vi "Get Set Operation.vi"(7 "Type":T1, 9 "String Operation":string, 11 "Numeric Operation":string) -> (2 "Operation":string)   [LabVIEW 2016]
uses:
  <vilib>/Utility/Data Type/Type Definitions/Data Type.ctl
  <vilib>/Utility/Data Type/NI_Data Type.lvlib
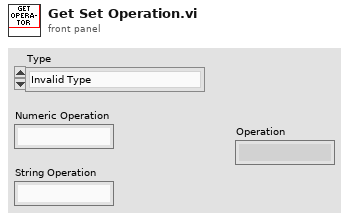
[diagram p1: front panel]
types:
  T1 = typedef "NI_Data Type.lvlib/Data Type.ctl" = enum8{"Invalid Type", "Void", "I8", "I16", "I32", "I64", "U8", "U16", "U32", "U64", "Single Float", "Double Float", "Extended Float", "Single Complex", "Double Complex", "Extended Complex", "Enum U8", "Enum U16", "Enum U32", "Enum U64", "Single Float With Unit", "Double Float With Unit", "Extended Float With Unit", "Single Complex with Unit", "Double Complex with Unit", "Extended Complex with Unit", "Boolean", "String", "Path", "Picture", "Tag", "Array", "Cluster", "Variant", "LV Variant", "Waveform", "Timestamp", "Digital Waveform", "Digital Data", "ExpressData", "Refnum", "External Data", "VI", "Poly VI", "LabVIEW Class Instance", "Fixed Point"}
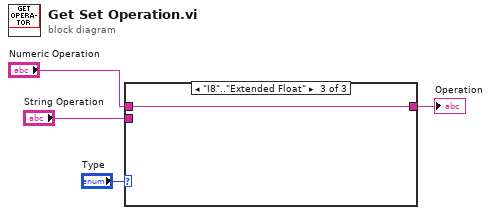
[diagram p0: block diagram]
diagram:
  n1 = case shown="\"I8\"..\"Extended Float\"" "Type" {
    tunnel: [_ w5 w6] -> w4
    tunnel: "Numeric Operation" -> [_ _ w6]
    tunnel: "String Operation" -> [_ w5 _]
    frame Default {
    }
    frame "String" {
    }
    frame "I8".."Extended Float" {
    }
  }
  "Operation" <- w4
